vi "Motion Profile Generator-Optimized.vi"(0 "Max Speed (rotations/sec)":dbl, 5 "Max Acceleration (rotations/sec^2)":dbl, 7 "Max Jerk (rotations/sec^3)":dbl, 9 "Rotations to Travel":dbl, 11 "Motion Profile Control Frame Rate":dbl) -> (4 "Position rotations":dbl[](array[numeric]), 6 "velocity rotations/sec":dbl[](array[numeric]))   [LabVIEW 2016]
panel:
  out "Waveform Chart":dbl[](graph)
  out "size(s)":i32
  out "Run Time (ms)":u32
  # "This is tempory and for testing purposes only"
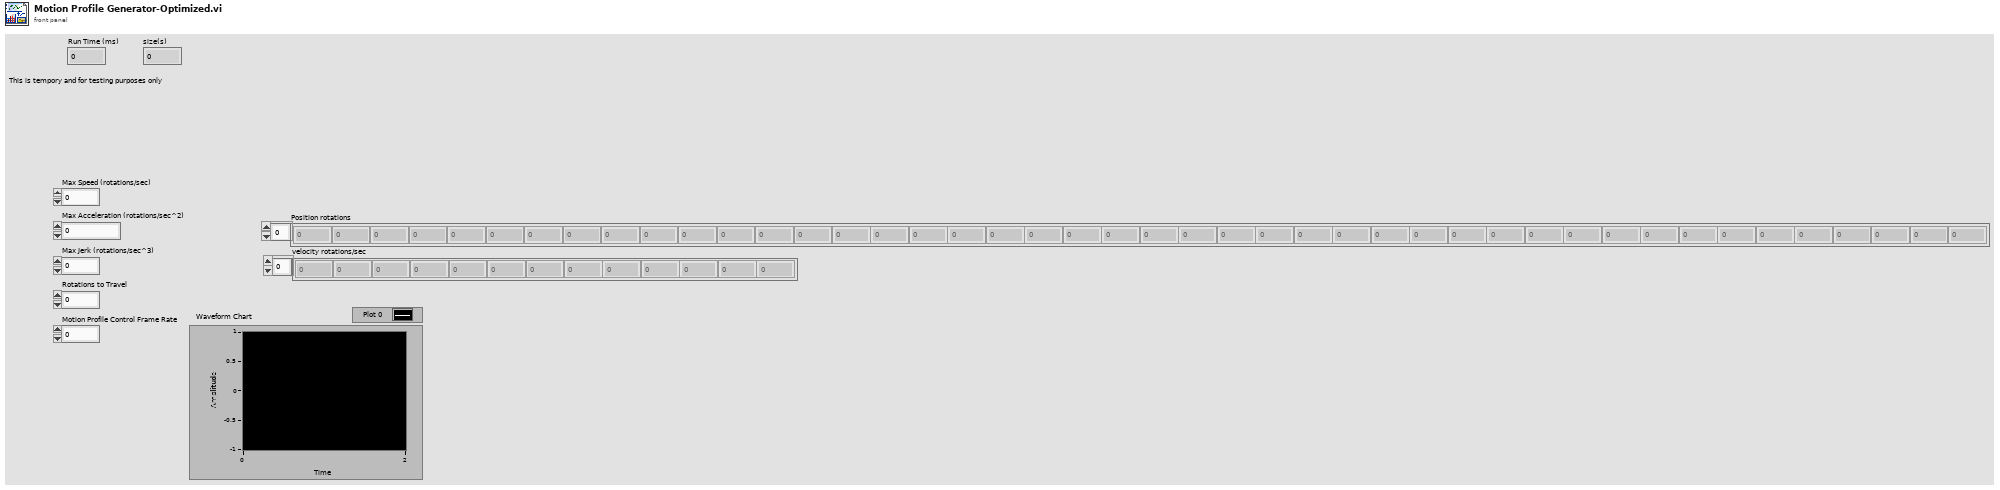
[diagram p1: front panel]
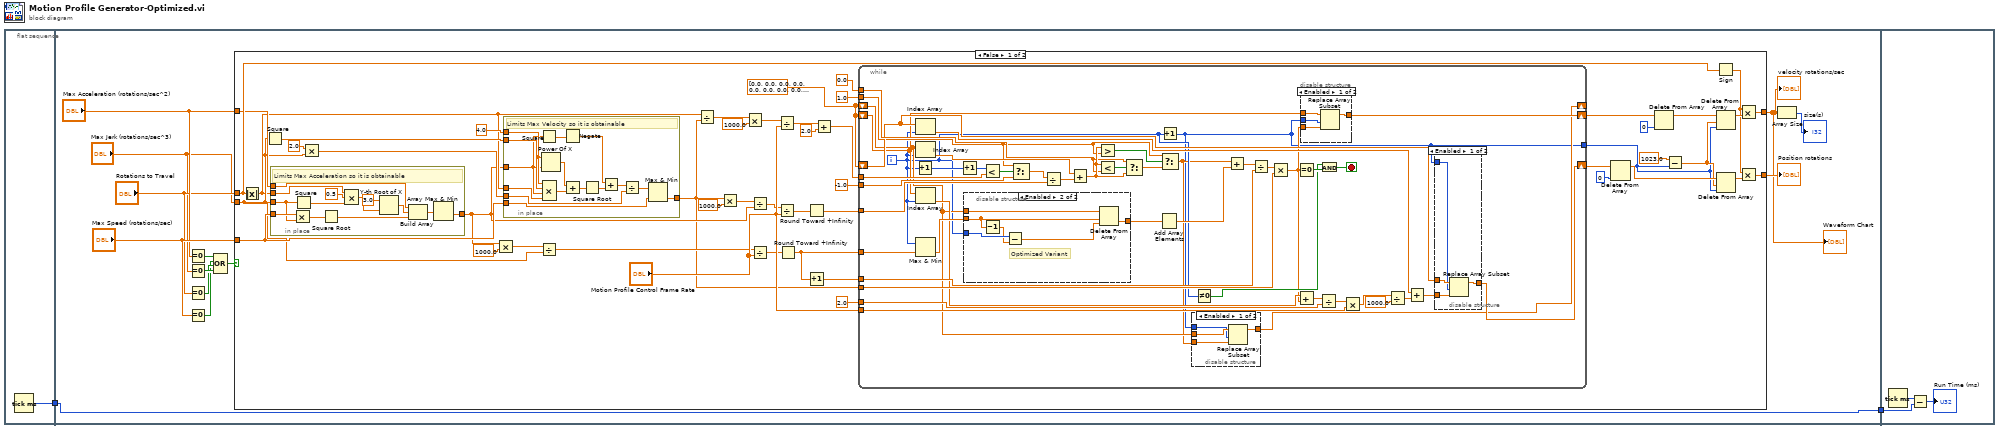
[diagram p0: block diagram]
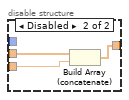
[diagram p2: hidden frame]
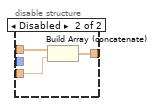
[diagram p3: hidden frame]
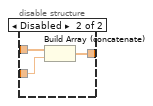
[diagram p4: hidden frame]
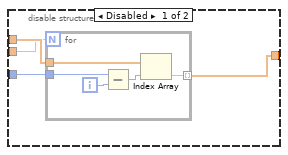
[diagram p5: hidden frame]
diagram:
  n1 = flat-sequence {
    tunnel: [w3] -> w1
    tunnel: [w7] -> w2
    tunnel: w1 -> [w7]
    tunnel: w2 -> [w175]
    frame #0 {
      n2 = Tick Count (ms)() -> (millisecond timer value=w3:u32)
    }
    frame #1 {
      n3 = Equal To 0?(x="Max Acceleration (rotations/sec^2)") -> (x = 0?=w16:bool)
      n4 = Equal To 0?(x="Max Jerk (rotations/sec^3)") -> (x = 0?=w11:bool)
      n5 = Equal To 0?(x="Rotations to Travel") -> (x = 0?=w10:bool)
      n6 = Equal To 0?(x="Max Speed (rotations/sec)") -> (x = 0?=w9:bool)
      n7 = Compound Arithmetic op=OR(w16, w9, w10, w11) -> (w8:bool)
      n8 = case shown="False" w8 {
        tunnel: "Max Acceleration (rotations/sec^2)" -> [w54 _]
        tunnel: "Max Speed (rotations/sec)" -> [w53 _]
        tunnel: "Max Jerk (rotations/sec^3)" -> [w52 _]
        tunnel: [w58 _] -> w4
        tunnel: [w57 _] -> w5
        tunnel: "Rotations to Travel" -> [w56 _]
        frame False {
          w17 = dbl[] [0.0, 0.0, 0.0, 0.0, 0.0, 0.0, 0.0, 0.0, 0.0, 0.0, 0.0, 0.0, 0.0, 0.0, 0.0, 0.0, 0.0, 0.0, 0.0, 0.0, 0.0, 0.0, 0.0, 0.0, 0.0, 0.0, 0.0, 0.0, 0.0, 0.0, 0.0, 0.0, 0.0, 0.0, 0.0, 0.0, 0.0, 0.0, 0.0, 0.0, 0.0, 0.0, 0.0, 0.0, 0.0, 0.0, 0.0, 0.0, 0.0, 0.0, 0.0, 0.0, 0.0, 0.0, 0.0, 0.0, 0.0, 0.0, 0.0, 0.0, 0.0, 0.0, 0.0, 0.0, 0.0, 0.0, 0.0, 0.0, 0.0, 0.0, 0.0, 0.0, 0.0, 0.0, 0.0, 0.0, 0.0, 0.0, 0.0, 0.0, 0.0, 0.0, 0.0, 0.0, 0.0, 0.0, 0.0, 0.0, 0.0, 0.0, 0.0, 0.0, 0.0, 0.0, 0.0, 0.0, 0.0, 0.0, 0.0, 0.0, 0.0, 0.0, 0.0, 0.0, 0.0, 0.0, 0.0, 0.0, 0.0, 0.0, 0.0, 0.0, 0.0, 0.0, 0.0, 0.0, 0.0, 0.0, 0.0, 0.0, 0.0, 0.0, 0.0, 0.0, 0.0, 0.0, 0.0, 0.0, 0.0, 0.0, 0.0, 0.0, 0.0, 0.0, 0.0, 0.0, 0.0, 0.0, 0.0, 0.0, 0.0, 0.0, 0.0, 0.0, 0.0, 0.0, 0.0, 0.0, 0.0, 0.0, 0.0, 0.0, 0.0, 0.0, 0.0, 0.0, 0.0, 0.0, 0.0, 0.0, 0.0, 0.0, 0.0, 0.0, 0.0, 0.0, 0.0, 0.0, 0.0, 0.0, 0.0, 0.0, 0.0, 0.0, 0.0, 0.0, 0.0, 0.0, 0.0, 0.0, 0.0, 0.0, 0.0, 0.0, 0.0, 0.0, 0.0, 0.0, 0.0, 0.0, 0.0, 0.0, 0.0, 0.0, 0.0, 0.0, 0.0, 0.0, 0.0, 0.0, 0.0, 0.0, 0.0, 0.0, 0.0, 0.0, 0.0, 0.0, 0.0, 0.0, 0.0, 0.0, 0.0, 0.0, 0.0, 0.0, 0.0, 0.0, 0.0, 0.0, 0.0, 0.0, 0.0, 0.0, 0.0, 0.0, 0.0, 0.0, 0.0, 0.0, 0.0, 0.0, 0.0, 0.0, 0.0, 0.0, 0.0, 0.0, 0.0, 0.0, 0.0, 0.0, 0.0, 0.0, 0.0, 0.0, 0.0, 0.0, 0.0, 0.0, 0.0, 0.0, 0.0, 0.0, 0.0, 0.0, 0.0, 0.0, 0.0, 0.0, 0.0, 0.0, 0.0, 0.0, 0.0, 0.0, 0.0, 0.0, 0.0, 0.0, 0.0, 0.0, 0.0, 0.0, 0.0, 0.0, 0.0, 0.0, 0.0, 0.0, 0.0, 0.0, 0.0, 0.0, 0.0, 0.0, 0.0, 0.0, 0.0, 0.0, 0.0, 0.0, 0.0, 0.0, 0.0, 0.0, 0.0, 0.0, 0.0, 0.0, 0.0, 0.0, 0.0, 0.0, 0.0, 0.0, 0.0, 0.0, 0.0, 0.0, 0.0, 0.0, 0.0, 0.0, 0.0, 0.0, 0.0, 0.0, 0.0, 0.0, 0.0, 0.0, 0.0, 0.0, 0.0, 0.0, 0.0, 0.0, 0.0, 0.0, 0.0, 0.0, 0.0, 0.0, 0.0, 0.0, 0.0, 0.0, 0.0, 0.0, 0.0, 0.0, 0.0, 0.0, 0.0, 0.0, 0.0, 0.0, 0.0, 0.0, 0.0, 0.0, 0.0, 0.0, 0.0, 0.0, 0.0, 0.0, 0.0, 0.0, 0.0, 0.0, 0.0, 0.0, 0.0, 0.0, 0.0, 0.0, 0.0, 0.0, 0.0, 0.0, 0.0, 0.0, 0.0, 0.0, 0.0, 0.0, 0.0, 0.0, 0.0, 0.0, 0.0, 0.0, 0.0, 0.0, 0.0, 0.0, 0.0, 0.0, 0.0, 0.0, 0.0, 0.0, 0.0, 0.0, 0.0, 0.0, 0.0, 0.0, 0.0, 0.0, 0.0, 0.0, 0.0, 0.0, 0.0, 0.0, 0.0, 0.0, 0.0, 0.0, 0.0, 0.0, 0.0, 0.0, 0.0, 0.0, 0.0, 0.0, 0.0, 0.0, 0.0, 0.0, 0.0, 0.0, 0.0, 0.0, 0.0, 0.0, 0.0, 0.0, 0.0, 0.0, 0.0, 0.0, 0.0, 0.0, 0.0, 0.0, 0.0, 0.0, 0.0, 0.0, 0.0, 0.0, 0.0, 0.0, 0.0, 0.0, 0.0, 0.0, 0.0, 0.0, 0.0, 0.0, 0.0, 0.0, 0.0, 0.0, 0.0, 0.0, 0.0, 0.0, 0.0, 0.0, 0.0, 0.0, 0.0, 0.0, 0.0, 0.0, 0.0, 0.0, 0.0, 0.0, 0.0, 0.0, 0.0, 0.0, 0.0, 0.0, 0.0, 0.0, 0.0, 0.0, 0.0, 0.0, 0.0, 0.0, 0.0, 0.0, 0.0, 0.0, 0.0, 0.0, 0.0, 0.0, 0.0, 0.0, 0.0, 0.0, 0.0, 0.0, 0.0, 0.0, 0.0, 0.0, 0.0, 0.0, 0.0, 0.0, 0.0, 0.0, 0.0, 0.0, 0.0, 0.0, 0.0, 0.0, 0.0, 0.0, 0.0, 0.0, 0.0, 0.0, 0.0, 0.0, 0.0, 0.0, 0.0, 0.0, 0.0, 0.0, 0.0, 0.0, 0.0, 0.0, 0.0, 0.0, 0.0, 0.0, 0.0, 0.0, 0.0, 0.0, 0.0, 0.0, 0.0, 0.0, 0.0, 0.0, 0.0, 0.0, 0.0, 0.0, 0.0, 0.0, 0.0, 0.0, 0.0, 0.0, 0.0, 0.0, 0.0, 0.0, 0.0, 0.0, 0.0, 0.0, 0.0, 0.0, 0.0, 0.0, 0.0, 0.0, 0.0, 0.0, 0.0, 0.0, 0.0, 0.0, 0.0, 0.0, 0.0, 0.0, 0.0, 0.0, 0.0, 0.0, 0.0, 0.0, 0.0, 0.0, 0.0, 0.0, 0.0, 0.0, 0.0, 0.0, 0.0, 0.0, 0.0, 0.0, 0.0, 0.0, 0.0, 0.0, 0.0, 0.0, 0.0, 0.0, 0.0, 0.0, 0.0, 0.0, 0.0, 0.0, 0.0, 0.0, 0.0, 0.0, 0.0, 0.0, 0.0, 0.0, 0.0, 0.0, 0.0, 0.0, 0.0, 0.0, 0.0, 0.0, 0.0, 0.0, 0.0, 0.0, 0.0, 0.0, 0.0, 0.0, 0.0, 0.0, 0.0, 0.0, 0.0, 0.0, 0.0, 0.0, 0.0, 0.0, 0.0, 0.0, 0.0, 0.0, 0.0, 0.0, 0.0, 0.0, 0.0, 0.0, 0.0, 0.0, 0.0, 0.0, 0.0, 0.0, 0.0, 0.0, 0.0, 0.0, 0.0, 0.0, 0.0, 0.0, 0.0, 0.0, 0.0, 0.0, 0.0, 0.0, 0.0, 0.0, 0.0, 0.0, 0.0, 0.0, 0.0, 0.0, 0.0, 0.0, 0.0, 0.0, 0.0, 0.0, 0.0, 0.0, 0.0, 0.0, 0.0, 0.0, 0.0, 0.0, 0.0, 0.0, 0.0, 0.0, 0.0, 0.0, 0.0, 0.0, 0.0, 0.0, 0.0, 0.0, 0.0, 0.0, 0.0, 0.0, 0.0, 0.0, 0.0, 0.0, 0.0, 0.0, 0.0, 0.0, 0.0, 0.0, 0.0, 0.0, 0.0, 0.0, 0.0, 0.0, 0.0, 0.0, 0.0, 0.0, 0.0, 0.0, 0.0, 0.0, 0.0, 0.0, 0.0, 0.0, 0.0, 0.0, 0.0, 0.0, 0.0, 0.0, 0.0, 0.0, 0.0, 0.0, 0.0, 0.0, 0.0, 0.0, 0.0, 0.0, 0.0, 0.0, 0.0, 0.0, 0.0, 0.0, 0.0, 0.0, 0.0, 0.0, 0.0, 0.0, 0.0, 0.0, 0.0, 0.0, 0.0, 0.0, 0.0, 0.0, 0.0, 0.0, 0.0, 0.0, 0.0, 0.0, 0.0, 0.0, 0.0, 0.0, 0.0, 0.0, 0.0, 0.0, 0.0, 0.0, 0.0, 0.0, 0.0, 0.0, 0.0, 0.0, 0.0, 0.0, 0.0, 0.0, 0.0, 0.0, 0.0, 0.0, 0.0, 0.0, 0.0, 0.0, 0.0, 0.0, 0.0, 0.0, 0.0, 0.0, 0.0, 0.0, 0.0, 0.0, 0.0, 0.0, 0.0, 0.0, 0.0, 0.0, 0.0, 0.0, 0.0, 0.0, 0.0, 0.0, 0.0, 0.0, 0.0, 0.0, 0.0, 0.0, 0.0, 0.0, 0.0, 0.0, 0.0, 0.0, 0.0, 0.0, 0.0, 0.0, 0.0, 0.0, 0.0, 0.0, 0.0, 0.0, 0.0, 0.0, 0.0, 0.0, 0.0, 0.0, 0.0, 0.0, 0.0, 0.0, 0.0, 0.0, 0.0, 0.0, 0.0, 0.0, 0.0, 0.0, 0.0, 0.0, 0.0, 0.0, 0.0, 0.0, 0.0, 0.0, 0.0, 0.0, 0.0, 0.0, 0.0, 0.0, 0.0, 0.0, 0.0, 0.0, 0.0, 0.0, 0.0, 0.0, 0.0, 0.0, 0.0, 0.0, 0.0, 0.0, 0.0, 0.0, 0.0, 0.0, 0.0, 0.0, 0.0, 0.0, 0.0, 0.0, 0.0, 0.0, 0.0, 0.0, 0.0, 0.0, 0.0, 0.0, 0.0, 0.0, 0.0, 0.0, 0.0, 0.0, 0.0, 0.0, 0.0, 0.0, 0.0, 0.0, 0.0, 0.0, 0.0, 0.0, 0.0, 0.0, 0.0, 0.0, 0.0, 0.0, 0.0, 0.0, 0.0, 0.0, 0.0, 0.0, 0.0, 0.0, 0.0, 0.0, 0.0, 0.0, 0.0, 0.0, 0.0, 0.0, 0.0, 0.0, 0.0, 0.0, 0.0, 0.0, 0.0, 0.0, 0.0, 0.0, 0.0, 0.0, 0.0, 0.0, 0.0, 0.0, 0.0, 0.0, 0.0, 0.0, 0.0, 0.0, 0.0, 0.0, 0.0, 0.0, 0.0, 0.0, 0.0, 0.0, 0.0, 0.0, 0.0, 0.0, 0.0, 0.0, 0.0, 0.0, 0.0, 0.0, 0.0, 0.0, 0.0, 0.0, 0.0, 0.0, 0.0, 0.0, 0.0, 0.0, 0.0, 0.0, 0.0, 0.0, 0.0, 0.0, 0.0, 0.0, 0.0, 0.0]
          n9 = Absolute Value(x=w56) -> (abs(x)=w36:dbl)
          n10 = Square(x=w52) -> (x^2=w39:dbl)
          n11 = in-place {
            in-place-border: w52 -> [w83]
            in-place-border: w54 -> [w87]
            in-place-border: [w80] -> w34
            in-place-border: w36 -> [w92]
            in-place-border: w53 -> [w84]
            # "Limits Max Acceleration so it is obtainable"
            n12 = Multiply(x=w84, y=w83) -> (x*y=w85:dbl)
            n13 = Square(x=w83) -> (x^2=w90:dbl)
            n14 = Square Root(x=w85) -> (sqrt(x)=w82:dbl)
            n15 = Compound Arithmetic op=MULTIPLY(w92, 0.5 ("value"), w90) -> (w89:dbl)
            n16 = Y-th Root of X(1:w89, 2:3.0 ("y")) -> (0:w86:dbl)
            n17 = Build Array(w87, w86, w82) -> (w81:dbl[])
            n18 = Array Max & Min(array=w81) -> (min value=w80:dbl)  [unwired: 3 out]
          }
          n19 = Multiply(x=2.0, y=w52) -> (x*y=w37:dbl)
          n20 = Multiply(x=w34, y=1000.0) -> (x*y=w35:dbl)
          n21 = in-place {
            in-place-border: w53 -> [w79]
            in-place-border: [w78] -> w31
            in-place-border: 4.0 ("x") -> [w74]
            in-place-border: w39 -> [w73]
            in-place-border: w37 -> [w67]
            in-place-border: w36 -> [w66]
            in-place-border: w34 -> [w65]
            # "Limits Max Velocity so it is obtainable"
            n22 = Square(x=w65) -> (x^2=w77:dbl)
            n23 = Power Of X(1:w65, 2:w74) -> (0:w75:dbl)
            n24 = Compound Arithmetic op=MULTIPLY(w74, w73, w65, w66) -> (w72:dbl)
            n25 = Negate(x=w77) -> (-x=w76:dbl)
            n26 = Add(x=w75, y=w72) -> (x+y=w71:dbl)
            n27 = Square Root(x=w71) -> (sqrt(x)=w70:dbl)
            n28 = Add(x=w76, y=w70) -> (x+y=w69:dbl)
            n29 = Divide(x=w69, y=w67) -> (x/y=w68:dbl)
            n30 = Max & Min(x=w68, y=w79) -> (min(x,y)=w78:dbl)  [unwired: 1 out]
          }
          n31 = Divide(x=w35, y=w52) -> (x/y=w42:dbl)
          n32 = Divide(x=w36, y=w31) -> (x/y=w28:dbl)
          n33 = Multiply(x=w31, y=1000.0) -> (x*y=w30:dbl)
          n34 = Multiply(x=w28, y=1000.0) -> (x*y=w27:dbl)
          n35 = Divide(x=w30, y=w34) -> (x/y=w44:dbl)
          n36 = Divide(x=w42, y="Motion Profile Control Frame Rate") -> (x/y=w41:dbl)
          n37 = Divide(x=w27, y="Motion Profile Control Frame Rate") -> (x/y=w46:dbl)
          n38 = Divide(x=w44, y="Motion Profile Control Frame Rate") -> (x/y=w43:dbl)
          n39 = Round Toward +Infinity(x=w41) -> (ceil(x): smallest int >= x=w62:dbl)
          n40 = Round Toward +Infinity(x=w43) -> (ceil(x): smallest int >= x=w63:dbl)
          n41 = Increment(x=w62) -> (x+1=w61:dbl)
          n42 = Add(x=w46, y=2.0) -> (x+y=w64:dbl)
          n43 = while {
            tunnel: w64 -> [w138]
            shift-right: [w100] -> _
            shift-left: w17 -> [w101]
            tunnel: w63 -> [w135]
            tunnel: w62 -> [w130]
            tunnel: w61 -> [w126]
            tunnel: w31 -> [w124]
            shift-right: [w102] -> w23
            shift-left: w17 -> [w104]
            shift-right: [w108] -> w25
            shift-left: w17 -> [w109]
            tunnel: "Motion Profile Control Frame Rate" -> [w116]
            tunnel: 1.0 ("t") -> [w105]
            tunnel: -1.0 ("f") -> [w112]
            tunnel: 0.0 ("y") -> [w111]
            tunnel: 2.0 ("y") -> [w110]
            tunnel: [w93] -> w18
            i -> [w99]
            stop <- w94 stop-if-true
            n44 = Increment(x=w99) -> (x+1=w132:i32)
            n45 = Index Array(array=w109, index=w99) -> (element=w121:dbl)
            n46 = Index Array(array=w101, index=w99) -> (element=w117:dbl)
            n47 = Index Array(array=w104, index=w99) -> (element=w120:dbl)
            n48 = Max & Min(x=w99, y=w130) -> (min(x,y)=w129:dbl)  [unwired: 1 out]
            n49 = Increment(x=w132) -> (x+1=w133:i32)
            n50 = disable-structure shown="Enabled" {
              disable-tunnel: w101 -> [w163 w174]
              disable-tunnel: w129 -> [w162 w170]
              disable-tunnel: w99 -> [w161 w173]
              disable-tunnel: [w160 w169] -> w106
              frame Disabled {
                n51 = for {
                  N: w162 -> [_]
                  tunnel: w161 -> [w167]
                  tunnel: w163 -> [w165]
                  tunnel: [w164] -> w160 mode=indexing
                  i -> [w168]
                  n52 = Subtract(x=w167, y=w168) -> (x-y=w166:i32)
                  n53 = Index Array(array=w165, index=w166) -> (element=w164:dbl)
                }
              }
              frame Enabled {
                # "Optimized Variant"
                n54 = Decrement(x=w170) -> (x-1=w172:dbl)
                n55 = Subtract(x=w173, y=w172) -> (x-y=w171:dbl)
                n56 = Delete From Array(array=w174, length=w170, index=w171) -> (deleted portion=w169:dbl[])  [unwired: 1 out]
              }
            }
            n57 = Less?(x=w133, y=w138) -> (x < y?=w137:bool)
            n58 = Select(t=w105, s=w137, f=w112) -> (s? t:f=w136:dbl)
            n59 = Divide(x=w136, y=w135) -> (x/y=w134:dbl)
            n60 = Add(x=w117, y=w134) -> (x+y=w131:dbl)
            n61 = Greater?(x=w131, y=w105) -> (0:w97:bool)
            n62 = Less?(x=w131, y=w111) -> (x < y?=w95:bool)
            n63 = Select(t=w111, s=w95, f=w131) -> (s? t:f=w96:dbl)
            n64 = Add Array Elements(numeric array=w106) -> (sum=w128:dbl)
            n65 = Increment(x=w99) -> (x+1=w93:i32)
            n66 = Select(t=w105, s=w97, f=w96) -> (s? t:f=w98:dbl)
            n67 = disable-structure shown="Enabled" {
              disable-tunnel: w101 -> [w142 w145]
              disable-tunnel: [w141 w143] -> w100
              disable-tunnel: w93 -> [w140 _]
              disable-tunnel: w98 -> [w139 w144]
              frame Enabled {
                n68 = Replace Array Subset(array=w142, new element=w139, index=w140) -> (w141:dbl[])
              }
              frame Disabled {
                n69 = Build Array (concatenate)(w145, w144) -> (w143:dbl[])
              }
            }
            n70 = Not Equal To 0?(x=w99) -> (x != 0?=w118:bool)
            n71 = Add(x=w98, y=w128) -> (x+y=w127:dbl)
            n72 = Divide(x=w127, y=w126) -> (x/y=w125:dbl)
            n73 = Multiply(x=w125, y=w124) -> (x*y=w103:dbl)
            n74 = Equal To 0?(x=w103) -> (x = 0?=w119:bool)
            n75 = Add(x=w120, y=w103) -> (x+y=w123:dbl)
            n76 = disable-structure shown="Enabled" {
              disable-tunnel: w104 -> [w149 w152]
              disable-tunnel: [w148 w150] -> w102
              disable-tunnel: w93 -> [w147 _]
              disable-tunnel: w103 -> [w146 w151]
              frame Enabled {
                n77 = Replace Array Subset(array=w149, new element=w146, index=w147) -> (w148:dbl[])
              }
              frame Disabled {
                n78 = Build Array (concatenate)(w152, w151) -> (w150:dbl[])
              }
            }
            n79 = Divide(x=w123, y=w110) -> (x/y=w122:dbl)
            n80 = And(x=w118, y=w119) -> (x .and. y?=w94:bool)
            n81 = Multiply(x=w122, y=w116) -> (x*y=w115:dbl)
            n82 = Divide(x=w115, y=1000.0) -> (x/y=w114:dbl)
            n83 = Add(x=w121, y=w114) -> (x+y=w107:dbl)
            n84 = disable-structure shown="Enabled" {
              disable-tunnel: w109 -> [w156 w159]
              disable-tunnel: [w155 w157] -> w108
              disable-tunnel: w93 -> [w154 _]
              disable-tunnel: w107 -> [w153 w158]
              frame Enabled {
                n85 = Replace Array Subset(array=w156, new element=w153, index=w154) -> (w155:dbl[])
              }
              frame Disabled {
                n86 = Build Array (concatenate)(w159, w158) -> (w157:dbl[])
              }
            }
          }
          n87 = Delete From Array(array=w25, index=0) -> (array with subset deleted=w24:dbl[])  [unwired: 1 in, 1 out]
          n88 = Delete From Array(array=w23, index=0) -> (array with subset deleted=w22:dbl[])  [unwired: 1 in, 1 out]
          n89 = Subtract(x=1023.0, y=w18) -> (x-y=w19:dbl)
          n90 = Sign(1:w56) -> (0:w55:dbl)
          n91 = Delete From Array(array=w22, length=w19, index=w18) -> (array with subset deleted=w59:dbl[])  [unwired: 1 out]
          n92 = Delete From Array(array=w24, length=w19, index=w18) -> (array with subset deleted=w60:dbl[])  [unwired: 1 out]
          n93 = Multiply(x=w55, y=w59) -> (x*y=w58:dbl[])
          n94 = Multiply(x=w55, y=w60) -> (x*y=w57:dbl[])
        }
        frame True {
        }
      }
      "velocity rotations/sec" <- w4
      "Position rotations" <- w5
      "Waveform Chart" <- w4
      n95 = Array Size(array=w4) -> (size(s)=→"size(s)":i32)
    }
    frame #2 {
      n96 = Tick Count (ms)() -> (millisecond timer value=w177:u32)
      n97 = Subtract(x=w177, y=w175) -> (x-y=→"Run Time (ms)":u32)
    }
  }
